vi "AlliGator Test Suite.vi"() -> ()   [LabVIEW 2021]
doc: "Runs a series of tests."
uses:
  AlliGator Q Element.ctl
  AlliGator Q Event.ctl
  AlliGator Action Engine.lvlib
  Files/AlliGator Files Tests.lvlib
panel:
  out "AlliGator Q out":refnum<queue>
  out "Error Out":errorcluster
  # "see the AlliGator License on the block diagram (Ctrl+E or Window:Show Block Diagram)"
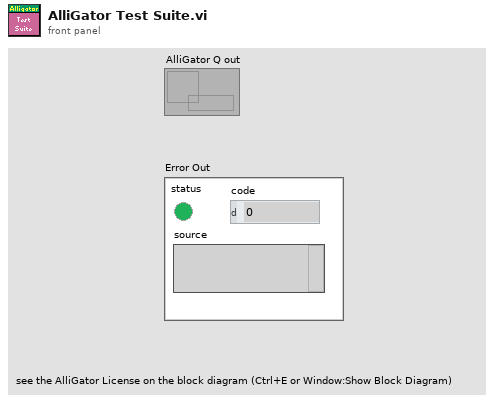
[diagram p1: front panel]
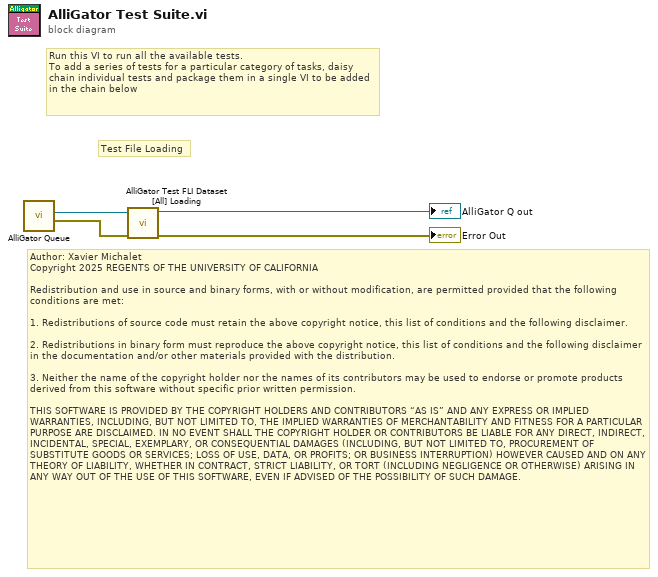
[diagram p0: block diagram]
diagram:
  # "Run this VI to run all the available tests.\nTo add a series of tests for a particular category of tasks, daisy chain individual tests and package them in a single VI to be added in the chain below"
  # "Test File Loading"
  # "Author: Xavier Michalet\nCopyright 2025 REGENTS OF THE UNIVERSITY OF CALIFORNIA\n\nRedistribution and use in source and binary forms, with or without modification, are permitted provided that the following conditions are met:\n\n1. Redistributions of source code must retain the above copyright notice, this list of conditions and the following disclaimer.\n\n2. Redistributions in binary form must reproduce the above copyright notice, this list of conditions and the following disclaimer in the documentation and/or other materials provided with the distribution.\n\n3. Neither the name of the copyright holder nor the names of its contributors may be used to endorse or promote products derived from this software without specific prior written permission.\n\nTHIS SOFTWARE IS PROVIDED BY THE COPYRIGHT HOLDERS AND CONTRIBUTORS “AS IS” AND ANY EXPRESS OR IMPLIED WARRANTIES, INCLUDING, BUT NOT LIMITED TO, THE IMPLIED WARRANTIES OF MERCHANTABILITY AND FITNESS FOR A PARTICULAR PURPOSE ARE DISCLAIMED. IN NO EVENT SHALL THE COPYRIGHT HOLDER OR CONTRIBUTORS BE LIABLE FOR ANY DIRECT, INDIRECT, INCIDENTAL, SPECIAL, EXEMPLARY, OR CONSEQUENTIAL DAMAGES (INCLUDING, BUT NOT LIMITED TO, PROCUREMENT OF SUBSTITUTE GOODS OR SERVICES; LOSS OF USE, DATA, OR PROFITS; OR BUSINESS INTERRUPTION) HOWEVER CAUSED AND ON ANY THEORY OF LIABILITY, WHETHER IN CONTRACT, STRICT LIABILITY, OR TORT (INCLUDING NEGLIGENCE OR OTHERWISE) ARISING IN ANY WAY OUT OF THE USE OF THIS SOFTWARE, EVEN IF ADVISED OF THE POSSIBILITY OF SUCH DAMAGE."
  n1 = call "AlliGator Queue.vi"() -> ("Error Out"=w4:errorcluster, "AlliGator Q"=w3:refnum<queue>)  [unwired: 8 in]
  n2 = call "AlliGator Test FLI Dataset [All] Loading.vi"("error in (no error)"=w4, "AlliGator Q in"=w3) -> ("error out"=→"Error Out":errorcluster, "AlliGator Q out"=→"AlliGator Q out":refnum<queue>)  [unwired: 8 in]
